vi "Window_plot.vi"() -> ()   [LabVIEW 2021]
doc: "This window has the capability to visualize and analyze the graphs of the stored signals from the Main_menu."
uses:
  <vilib>/Waveform/WDTOps.llb/WDT Get Waveform Subset DBL.vi
panel:
  in  "Slide Offset":u32(slide) scale=0.0..10.0
  in  "Select offset":string(combo)
  out "Waveform Graph":waveform(dbl)[](graph) caption="Waveform Graph 2"
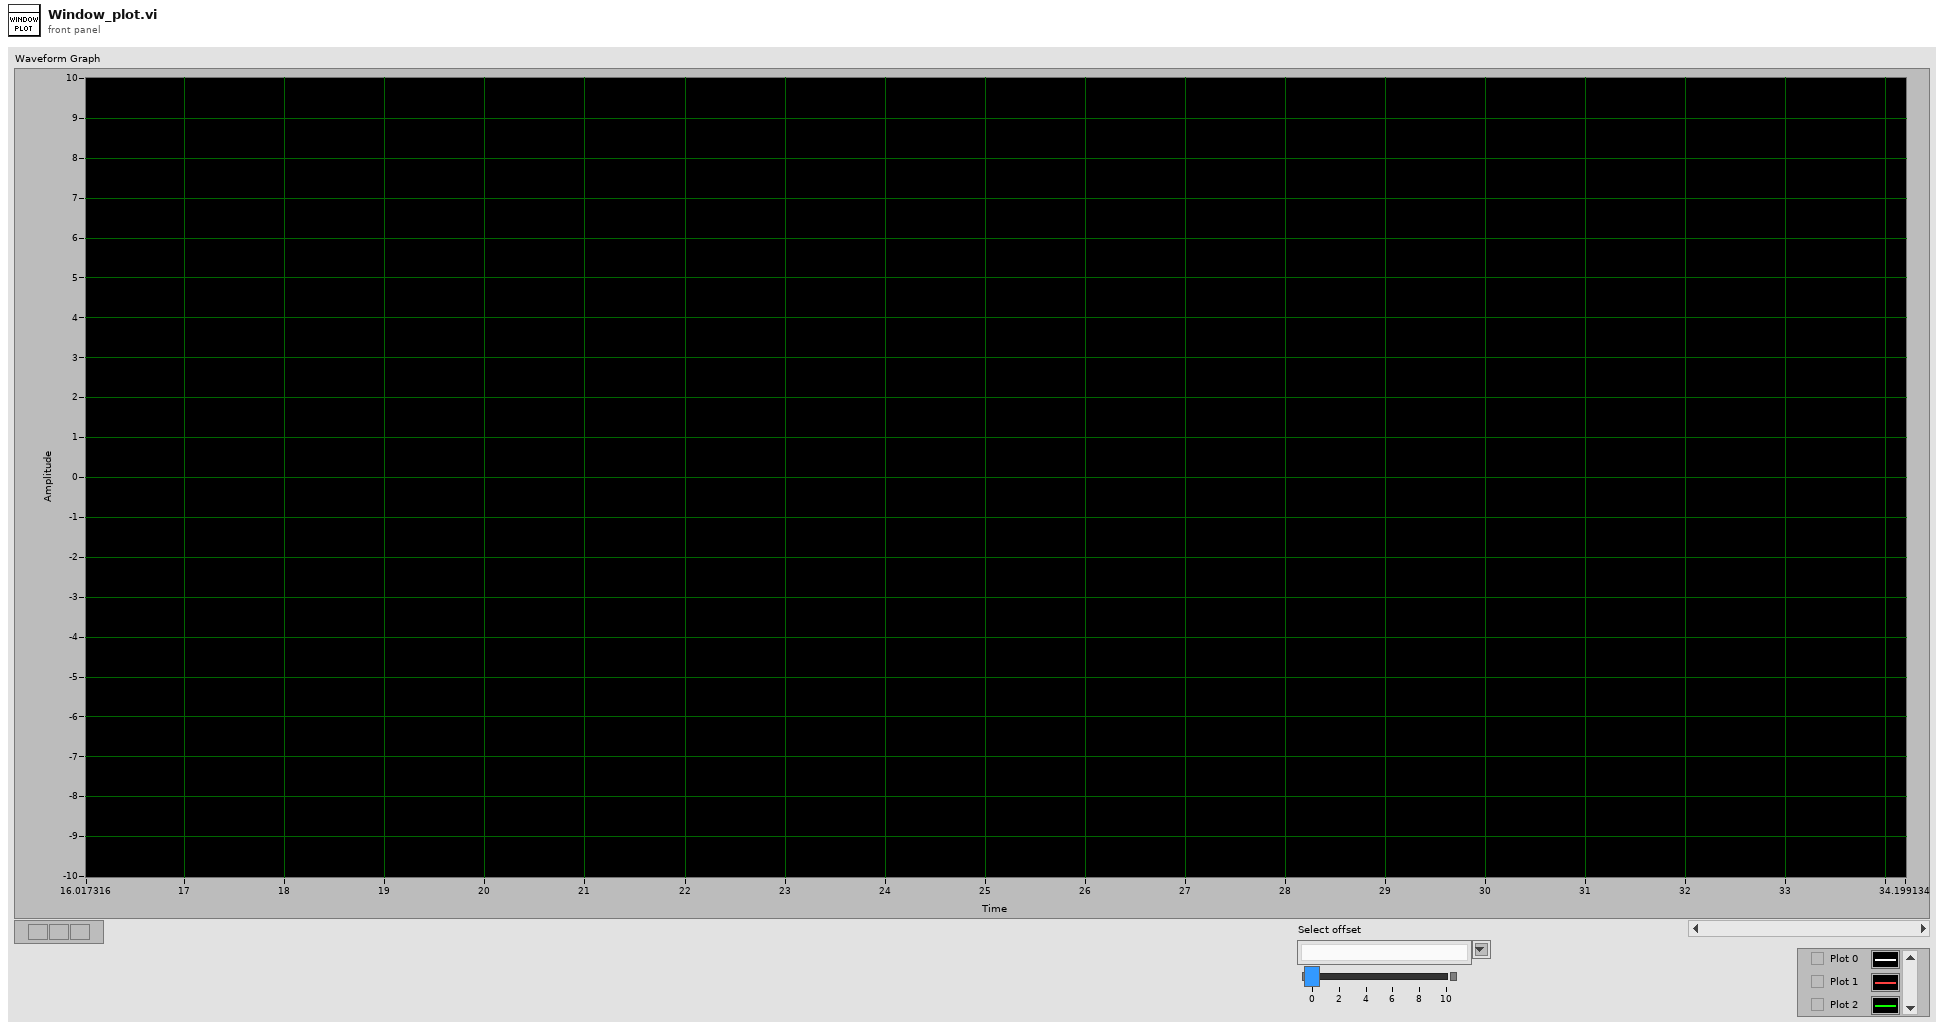
[diagram p1: front panel]
types:
  T1 = cluster{"Mode signal_Global":refnum<vi>, "Trace name":refnum<vi>, "Execution:State":refnum<vi>, "message":refnum<vi>, "Filename":refnum<vi>, "Closed w":refnum<vi>, "total \nrefresh time":refnum<vi>, "Mode signal_Global 2":string, "Filename 2":string, "Execution:State 2":enum32{"Bad", "Idle", "Run top level", "Running"}, "message 2":string, "Trace name 2":string, "total \nrefresh time 2":i32, "refresh time 2":i32, "Continous":bool}
  T2 = cluster{"plot Names":string[], "Waveforms arrays":waveform(dbl)[], "signals_HW":string[][], "Waveforms arrays csv":waveform(dbl)[], "signals_csv":string[], "Signals_name":string[], "Mode_signal_conf":u8, "Request_plots_array":cluster{string, waveform(dbl)}[], "time out":i32, " global r time":u32, "Refresh time":u32, "Local Mode":enum32{"Resume", "Hold"}}
  T3 = enum32{"Invalid", "Standard", "Closed", "Hidden", "Minimized", "Maximized"}
  T4 = enum32{"Bad", "Idle", "Run top level", "Running"}
  T5 = cluster{"plot Names":string[], "Waveforms arrays":waveform(dbl)[], "signals_HW":string[][], "Waveforms arrays csv":waveform(dbl)[], "signals_csv":string[], "Signals_name":string[], "Mode_signal_conf":u8, "Request_plots_array":cluster{string, "Waveform":waveform(dbl)}[], "time out":i32, " global r time":u32, "Refresh time":u32, "Local Mode":enum32{"Resume", "Hold"}}
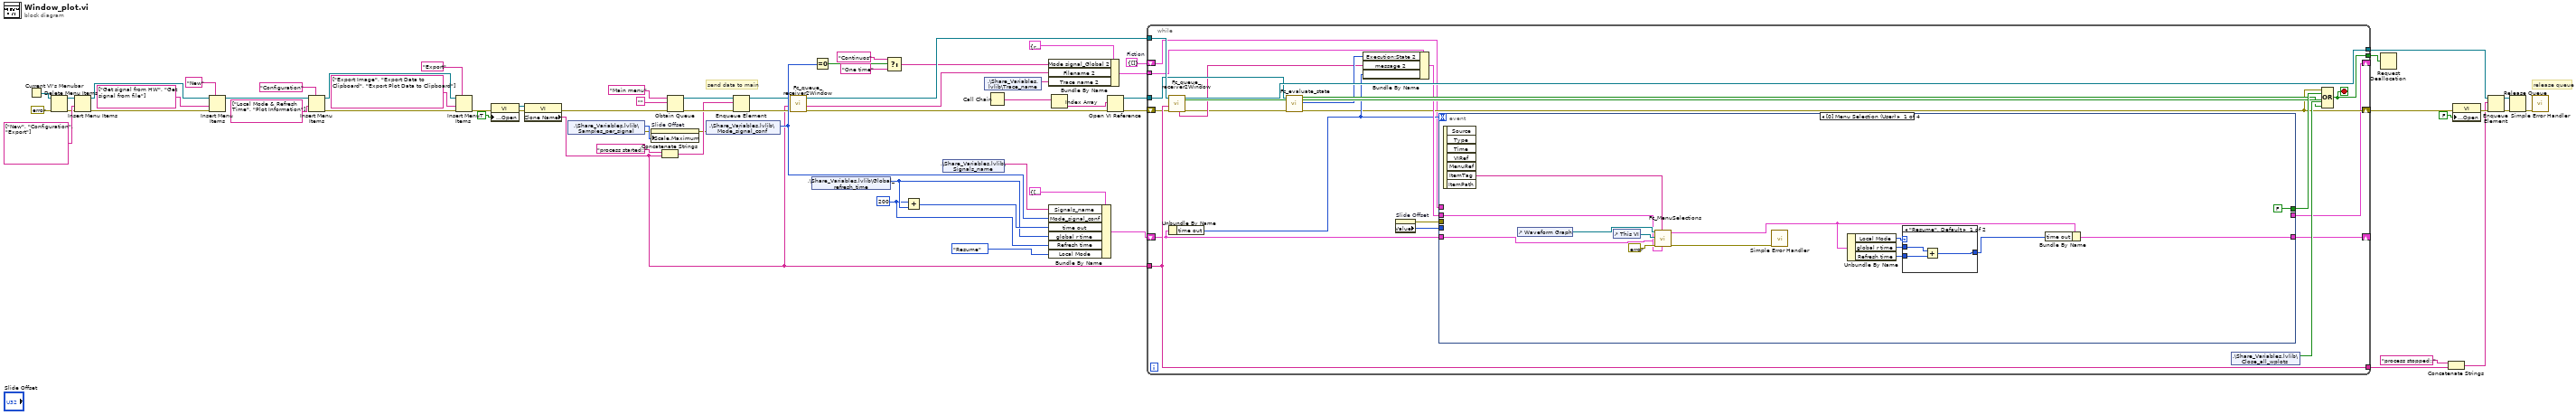
[diagram p0: block diagram]
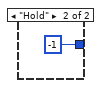
[diagram p2: hidden frame]
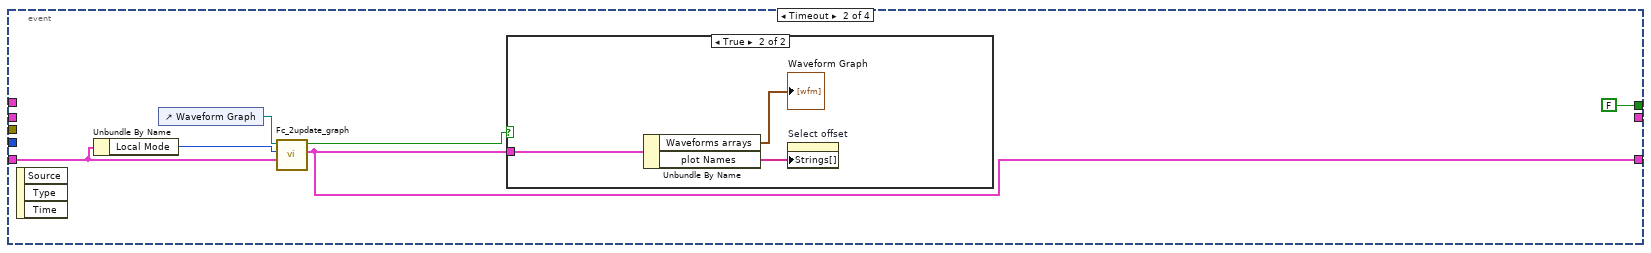
[diagram p3: hidden frame]
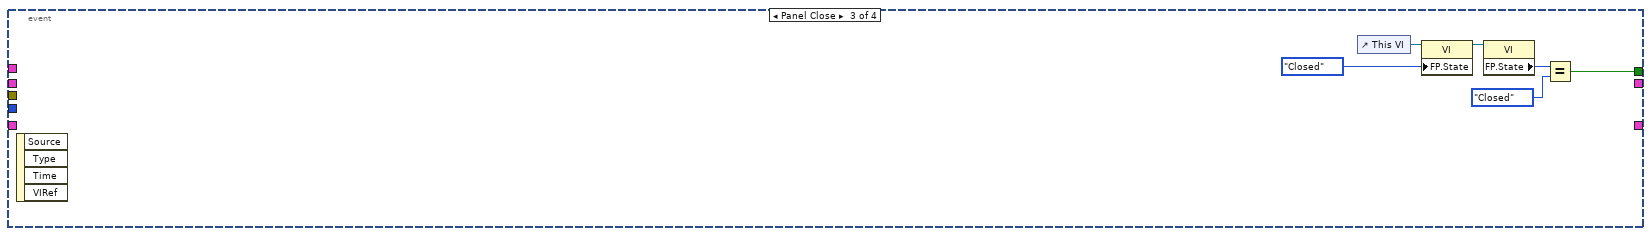
[diagram p5: hidden frame]
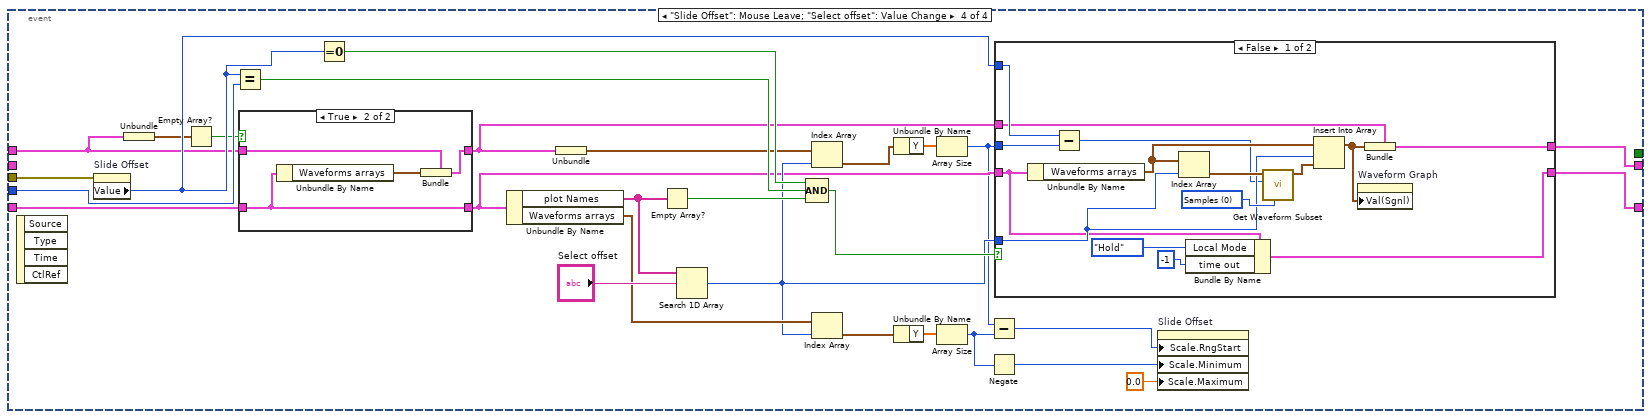
[diagram p6: hidden frame]
diagram:
  w2 = cluster{"Fiction Wavef":waveform(dbl)[]} {"Fiction Wavef"=[]}  # Fiction
  w31 = u32 200 ("Refresh time")
  # "send data to main"
  # "release queue"
  n1 = Current VI's Menubar() -> (w20:refnum<k9>)
  n2 = Delete Menu Items(6:errorcluster {"status"=FALSE, "code"=0, "source"=""} ("error in (no error)"), 9:w20) -> (0:w19:errorcluster, 3:w18:refnum<k9>)  [unwired: 2 in]
  n3 = Insert Menu Items(6:w19, 7:string[] ["New", "Configuration", "Export"], 9:w18) -> (0:w25:errorcluster, 3:w24:refnum<k9>)  [unwired: 3 in, 1 out]
  n4 = Insert Menu Items(5:"New", 6:w25, 7:string[] ["Get signal from HW", "Get signal from file"], 9:w24) -> (3:w13:refnum<k9>)  [unwired: 2 in, 2 out]
  n5 = Insert Menu Items(5:"Configuration" ("menu tag"), 7:string[] ["Local Mode & Refresh Time", "Plot Information"] ("item tags"), 9:w13) -> (0:w9:errorcluster, 3:w12:refnum<k9>)  [unwired: 3 in, 1 out]
  n6 = Insert Menu Items(5:"Export" ("menu tag"), 6:w9, 7:string[] ["Export Image", "Export Data to Clipboard", "Export Plot Data to Clipboard"], 9:w12) -> (0:w26:errorcluster)  [unwired: 2 in, 2 out]
  n7 = property class="VI"(error in=w26, "Front Panel.Open"=TRUE ("Front Panel Window:Open")) -> (reference out=w51:refnum<vi>, error out=w61:errorcluster)  [unwired: 1 in]
  n8 = property class="VI"(reference=w51, error in=w61) -> (error out=w44:errorcluster, "Clone Name"=w34:string)  [unwired: 1 out]
  n9 = shared-variable ".\\Share_Variables.lvlib\\Samples_per_signal"() -> (w6:u32, error out=w5:errorcluster)  [unwired: 1 in]
  n10 = property on="Slide Offset" class="Slide (strict)"(error in=w5, "Scale.Maximum"=w6) -> (error out=w3:errorcluster)  [unwired: 1 in, 1 out]
  n11 = Concatenate Strings("process started::" ("name (unnamed)"), w34) -> (w62:string)
  n12 = Obtain Queue(name (unnamed)="Main menu", element data type="", error in (no error)=w44) -> (queue out=w64:refnum<queue>, error out=w63:errorcluster)  [unwired: 2 in, 1 out]
  n13 = shared-variable ".\\Share_Variables.lvlib\\Mode_signal_conf"(error in=w3) -> (w45:u8)  [unwired: 1 out]
  n14 = Enqueue Element(queue=w64, element=w62, error in (no error)=w63) -> (queue out=w37:refnum<queue>, error out=w35:errorcluster)  [unwired: 1 in, 1 out]
  n15 = call "Fc_queue_receiver2Window.vi"("error in (no error)"=w35, "Clone Name"=w34, "Queue in"=w37) -> ("error out"=w4:errorcluster, "Filename"=w32:string, "Queue out"=w36:refnum<queue>)  [unwired: 4 in, 2 out]
  n16 = shared-variable ".\\Share_Variables.lvlib\\Global_refresh_time"() -> (w40:u16)  [unwired: 1 in, 1 out]
  n17 = Equal To 0?(x=w45) -> (x = 0?=w8:bool)
  n18 = Select(t="Continuos", s=w8, f="One time") -> (s? t:f=w33:string)
  n19 = Add(x=w31, y=w40) -> (x+y=w41:u32)
  n20 = shared-variable ".\\Share_Variables.lvlib\\Signals_name"() -> (w46:string[])  [unwired: 1 in, 1 out]
  n21 = shared-variable ".\\Share_Variables.lvlib\\Trace_name"() -> (w30:string)  [unwired: 1 in, 1 out]
  n22 = Call Chain() -> (call chain=w50:string[])
  n23 = Bundle By Name(cluster=T1 {"Mode signal_Global"=refnum, "Trace name"=refnum, "Execution:State"=refnum, "message"=refnum, "Filename"=refnum, "Closed w"=refnum, "total \nrefresh time"=refnum, "Mode signal_Global 2"="", "Filename 2"="", "Execution:State 2"=enum."Idle", "message 2"="", "Trace name 2"="", "total \nrefresh time 2"=0, "refresh time 2"=0, "Continous"=TRUE}, "Mode signal_Global 2"=w33, "Filename 2"=w32, "Trace name 2"=w30) -> (w39:T1)
  n24 = Bundle By Name(cluster=T2 {"plot Names"=[], "Waveforms arrays"=[], "signals_HW"=[], "Waveforms arrays csv"=[], "signals_csv"=[], "Signals_name"=[], "Mode_signal_conf"=0, "Request_plots_array"=[], "time out"=300, " global r time"=0, "Refresh time"=0, "Local Mode"=enum."Resume"}, "Signals_name"=w46, "Mode_signal_conf"=w45, "time out"=w41, "global r time"=w40, "Refresh time"=w31, "Local Mode"=enum32{"Resume", "Hold"}."Resume") -> (w47:T2)
  n25 = Index Array(array=w50) -> (element=w49:string)  [unwired: 1 in]
  n26 = Open VI Reference(vi path=w49, error in (no error)=w4) -> (vi reference=w48:refnum<vi>, error out=w28:errorcluster)  [unwired: 4 in]
  n27 = while {
    tunnel: w36 -> [w90]
    tunnel: [w89] -> w60
    shift-right: [w72] -> w55
    shift-left: w28 -> [w79]
    tunnel: [w84] -> w53
    tunnel: w48 -> [w82]
    tunnel: w34 -> [w84]
    shift-right: [w85] -> _
    shift-left: w47 -> [w83]
    tunnel: [w81] -> w43
    tunnel: w39 -> [w78]
    shift-right: [w68] -> _
    shift-left: w2 -> [w69]
    stop <- w81 stop-if-true
    n28 = call "Fc_queue_receiver2Window.vi"("error in (no error)"=w79, "Clone Name"=w84, "Queue in"=w90) -> ("error out"=w73:errorcluster, "Queue out"=w89:refnum<queue>, "message"=w75:string, "Stop"=w87:bool)  [unwired: 4 in, 1 out]
    n29 = Unbundle By Name(w83) -> ("time out"=w74:i32)
    n30 = call "Fc_evaluate_state.vi"("error in (no error)"=w73, "VI in"=w82) -> ("error out"=w72:errorcluster, "Exec.State"=w77:T4, "Status out"=w80:bool)  [unwired: 7 in]
    n31 = Bundle By Name(cluster=w78, "Execution:State 2"=w77, "message 2"=w75, "total \nrefresh time 2"=w74) -> (w76:T1)
    n32 = property on="Slide Offset" class="Slide (strict)"() -> (error out=w71:errorcluster, "Value"=w70:u32)  [unwired: 2 in, 1 out]
    n33 = event shown="[0] Menu Selection (User)" {
      selector: _ -> [_ _ _ _]
      dyn-events: _ -> [_ _ _ _]
      timeout: w74 -> [_ _ _ _]
      tunnel: [FALSE FALSE w121 _] -> w88
      tunnel: [w91 w109 _ w142] -> w85
      tunnel: w83 -> [w96 w111 _ w144]
      tunnel: w76 -> [w98 _ _ _]
      tunnel: w71 -> [_ _ _ w152]
      tunnel: w70 -> [_ _ _ w150]
      tunnel: w69 -> [_ _ _ w127]
      tunnel: [_ _ _ w124] -> w68
      event Menu Selection (User) {
        n34 = event-data() -> ("ItemTag"=w104:string)  [unwired: 1 in, 6 out]
        n35 = control-ref of="Waveform Graph"() -> (w100:refnum<vi>)
        n36 = control-ref of="This VI"() -> (w99:refnum<vi>)
        n37 = call "Fc_MenuSelections.vi"("Cluster References"=w98, "ItemTag"=w104, "error in (no error)"=errorcluster {"status"=FALSE, "code"=0, "source"=""}, "Cluster in"=w96, "VI caller"=w99, "WaveformGraph in"=w100) -> ("error out"=w102:errorcluster, "Cluster out"=w92:T5)  [unwired: 4 in]
        n38 = call <vilib>:"Simple Error Handler.vi"("error in (no error)"=w102) -> ()  [unwired: 4 in, 5 out]
        n39 = Unbundle By Name(w92) -> ("Local Mode"=w95:enum32{"Resume", "Hold"}, "global r time"=w94:u32, "Refresh time"=w93:u32)
        n40 = case shown="\"Resume\", Default" w95 {
          tunnel: [w105 -1 ("time out")] -> w97
          tunnel: w94 -> [w107 _]
          tunnel: w93 -> [w106 _]
          frame "Resume", Default {
            n41 = Add(x=w107, y=w106) -> (x+y=w105:u32)
          }
          frame "Hold" {
          }
        }
        n42 = Bundle By Name(cluster=w92, "time out"=w97) -> (w91:T5)
      }
      event Timeout {
        n43 = event-data() -> ()  [unwired: 1 in, 3 out]
        n44 = Unbundle By Name(w111) -> ("Local Mode"=w110:enum32{"Resume", "Hold"})
        n45 = control-ref of="Waveform Graph"() -> (w112:refnum<vi>)
        n46 = call "Fc_2update_graph.vi"("Cluster in"=w111, "Local Mode"=w110, "WaveformGraph in"=w112) -> ("Cluster in 2"=w109:T5, "Update Waveform Graph"=w113:bool)  [unwired: 7 in]
        n47 = case shown="True" w113 {
          tunnel: w109 -> [_ w116]
          frame False {
          }
          frame True {
            n48 = Unbundle By Name(w116) -> ("Waveforms arrays"=→"Waveform Graph":waveform(dbl)[], "plot Names"=w115:string[])
            n49 = property on="Select offset" class="CmbBox"("Strings[]"=w115) -> ()  [unwired: 2 in, 2 out]
          }
        }
      }
      event Panel Close {
        n50 = event-data() -> ()  [unwired: 1 in, 4 out]
        n51 = control-ref of="This VI"() -> (w120:refnum<vi>)
        n52 = property class="VI"(reference=w120, "FP.State"=T3."Closed" ("Front Panel Window:State")) -> (reference out=w118:refnum<vi>)  [unwired: 1 in, 1 out]
        n53 = property class="VI"(reference=w118) -> ("FP.State"=w122:T3)  [unwired: 1 in, 2 out]
        n54 = Equal?(x=w122, y=T3."Closed" ("Front Panel Window:State")) -> (x = y?=w121:bool)
      }
      event "Slide Offset": Mouse Leave; "Select offset": Value Change {
        n55 = event-data() -> ()  [unwired: 1 in, 4 out]
        n56 = property on="Slide Offset" class="Slide (strict)"(error in=w152) -> ("Value"=w143:u32)  [unwired: 1 in, 2 out]
        n57 = Unbundle(w127) -> ("Fiction Wavef"=w128:waveform(dbl)[])
        n58 = Empty Array?(array=w128) -> (empty?=w131:bool)
        n59 = Equal?(x=w143, y=w150) -> (x = y?=w148:bool)
        n60 = case shown="True" w131 {
          tunnel: w144 -> [w154 w158]
          tunnel: [w154 w158] -> w130
          tunnel: w127 -> [w153 w156]
          tunnel: [w153 w155] -> w125
          frame False {
          }
          frame True {
            n61 = Unbundle By Name(w158) -> ("Waveforms arrays"=w157:waveform(dbl)[])
            n62 = Bundle(cluster=w156, "Fiction Wavef"=w157) -> (w155:cluster{"Fiction Wavef":waveform(dbl)[]})
          }
        }
        n63 = Equal To 0?(x=w143) -> (x = 0?=w149:bool)
        n64 = Unbundle By Name(w130) -> ("plot Names"=w145:string[], "Waveforms arrays"=w140:waveform(dbl)[])
        n65 = Unbundle(w125) -> ("Fiction Wavef"=w126:waveform(dbl)[])
        n66 = Empty Array?(array=w145) -> (empty?=w147:bool)
        n67 = Search 1D Array(1D array=w145, element="Select offset") -> (index of element=w136:i32)  [unwired: 1 in]
        n68 = Compound Arithmetic op=AND(w149, w148, w147) -> (w146:bool)
        n69 = Index Array(array=w126, index=w136) -> (element=w135:waveform(dbl))
        n70 = Index Array(array=w140, index=w136) -> (element=w139:waveform(dbl))
        n71 = Unbundle By Name(w135) -> ("Y"=w134:dbl[])
        n72 = Unbundle By Name(w139) -> ("Y"=w141:dbl[])
        n73 = Array Size(array=w134) -> (size(s)=w129:i32)
        n74 = Array Size(array=w141) -> (size(s)=w133:i32)
        n75 = Subtract(x=w129, y=w133) -> (x-y=w132:i32)
        n76 = Negate(x=w133) -> (-x=w137:i32)
        n77 = case shown="False" w146 {
          tunnel: w130 -> [w165 w175]
          tunnel: w136 -> [w166 _]
          tunnel: w143 -> [w164 _]
          tunnel: [w169 w175] -> w142
          tunnel: w129 -> [w163 _]
          tunnel: w125 -> [w161 w174]
          tunnel: [w159 w174] -> w124
          frame False {
            w173 = u16 0 items=["Samples", "Relative Time"] ("start/duration format")
            n78 = Unbundle By Name(w165) -> ("Waveforms arrays"=w171:waveform(dbl)[])
            n79 = Subtract(x=w164, y=w163) -> (x-y=w162:u32)
            n80 = Index Array(array=w171, index=w166) -> (element=w172:waveform(dbl))
            n81 = Bundle By Name(cluster=w165, "Local Mode"=enum32{"Resume", "Hold"}."Hold", "time out"=-1) -> (w169:T2)
            n82 = call-poly <vilib>:"Get Waveform Subset.vi"("start/duration format"=w173, "start samples/time"=w162, "waveform in"=w172) -> ("waveform out"=w170:waveform(dbl))  [unwired: 3 in, 3 out]
            n83 = Insert Into Array(array=w171, index=w166, new element=w170) -> (w160:waveform(dbl)[])
            n84 = property on="Waveform Graph" class="WFGraph (strict)"("Val(Sgnl)"=w160) -> ()  [unwired: 2 in, 2 out]
            n85 = Bundle(cluster=w161, "Fiction Wavef"=w160) -> (w159:cluster{"Fiction Wavef":waveform(dbl)[]})
          }
          frame True {
          }
        }
        n86 = property on="Slide Offset" class="Slide (strict)"("Scale.RngStart"=w132, "Scale.Minimum"=w137, "Scale.Maximum"=0.0 ("Scale.Range:Minimum")) -> ()  [unwired: 2 in, 2 out]
      }
    }
    n87 = shared-variable ".\\Share_Variables.lvlib\\Close_all_wplots"() -> (w86:bool)  [unwired: 1 in, 1 out]
    n88 = Compound Arithmetic op=OR(w72, w88, w87, w86, w80) -> (w81:bool)
  }
  n89 = Request Deallocation(w43) -> ()
  n90 = Concatenate Strings("process stopped::" ("string"), w53) -> (w52:string)
  n91 = property class="VI"(error in=w55, "Front Panel.Open"=FALSE ("Front Panel Window:Open")) -> (error out=w57:errorcluster)  [unwired: 1 in, 1 out]
  n92 = Enqueue Element(queue=w60, element=w52, error in (no error)=w57) -> (queue out=w59:refnum<queue>, error out=w58:errorcluster)  [unwired: 1 in, 1 out]
  n93 = Release Queue(queue=w59, error in (no error)=w58) -> (error out=w29:errorcluster)  [unwired: 1 in, 2 out]
  n94 = call <vilib>:"Simple Error Handler.vi"("error in (no error)"=w29) -> ()  [unwired: 4 in, 5 out]
